vi "Measure NPLC.vi"(6 "NPLC (1.000)":dbl=1.0, 8 "error in (no error)":errorcluster, 9 "Channel (Channel A)":T1, 10 "Node In":string, 11 "VISA resource name":refnum<visa-resource-name>) -> (0 "error out":errorcluster, 2 "Node Out":string, 3 "VISA resource name out":refnum<visa-resource-name>, 4 "Command String":string)   [LabVIEW 2009, in "Keithley 2600 Series.lvlib"]
doc: "This VI sets the integration aperture for measurements. When used with 265x instruments, this attribute is disabled when the Fast ADC is selected in the Measure ADC vi.\n\n<b>Functions and Attributes Used</b>\nsmuX.measure.nplc"
uses:
  <instrlib>/Keithley 2600 Series/Keithley 2600 Series.lvlib
  <instrlib>/Keithley 2600 Series/Public/Channel.ctl
  <instrlib>/Keithley 2600 Series/Private/GlobalVariables.vi
panel:
  # "(c) 2008 Keithley Instruments, Inc.  ALL RIGHTS RESERVED."
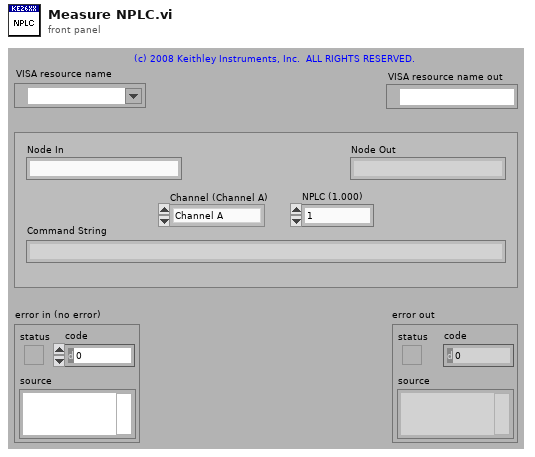
[diagram p1: front panel]
types:
  T1 = typedef "Keithley 2600 Series.lvlib/Channel.ctl" = enum32{"Channel A", "Channel B"}
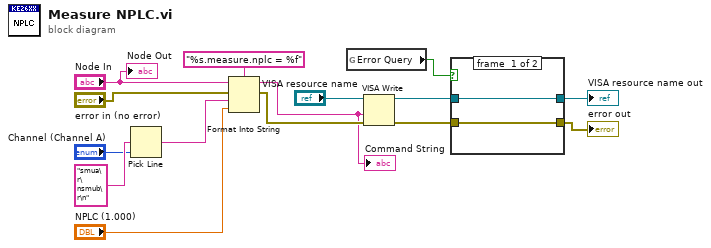
[diagram p0: block diagram]
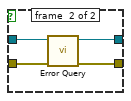
[diagram p2: hidden frame]
diagram:
  n1 = Pick Line(multi-line string="smua\r\nsmub\r\n" ("options"), line index="Channel (Channel A)") -> (output string=w5:string)  [unwired: 1 out]
  n2 = Format Into String(format string="%s.measure.nplc = %f", initial string="Node In", error in="error in (no error)", w5, "NPLC (1.000)") -> (resulting string=w1:string, error out=w2:errorcluster)
  "Command String" <- w1
  n3 = global read "GlobalVariables.vi" "Error Query"() -> (w13:bool)
  n4 = VISA Write(VISA resource name="VISA resource name", write buffer=w1, error in (no error)=w2) -> (VISA resource name out=w12:refnum<visa-resource-name>, error out=w11:errorcluster)  [unwired: 1 out]
  n5 = case shown="True" w13 {
    tunnel: w12 -> [w17 w21]
    tunnel: w11 -> [w16 w20]
    tunnel: [w17 w19] -> w9
    tunnel: [w16 w18] -> w10
    frame #0 {
    }
    frame #1 {
      n6 = call <instrlib>:"Error Query.vi"("error in (no error)"=w20, "VISA resource name"=w21) -> ("error out"=w18:errorcluster, "VISA resource name out"=w19:refnum<visa-resource-name>)  [unwired: 8 out]
    }
  }
  "VISA resource name out" <- w9
  "error out" <- w10
  "Node Out" <- "Node In"
